vi "Constants.vi"() -> ()   [LabVIEW 2019, in "Reset Hardware Shared.lvlib"]
doc: "Use this Global VI to access the GUIDs assigned to the page resources of the Custom Device."
uses:
  Reset Hardware Shared.lvlib
panel:
  in  "Tab Control":enum32{"GUIDs", "Constants", "Properties"}(tab)
  in  "Reset Hardware":string="5e0dd9d5-b0d1-4b33-abc2-5f3c1ff7365d"
  in  "Reset XNET":string
  in  "Reset DAQmx AO":string
  in  "Compiled.Settings":string="Compiled.Settings"
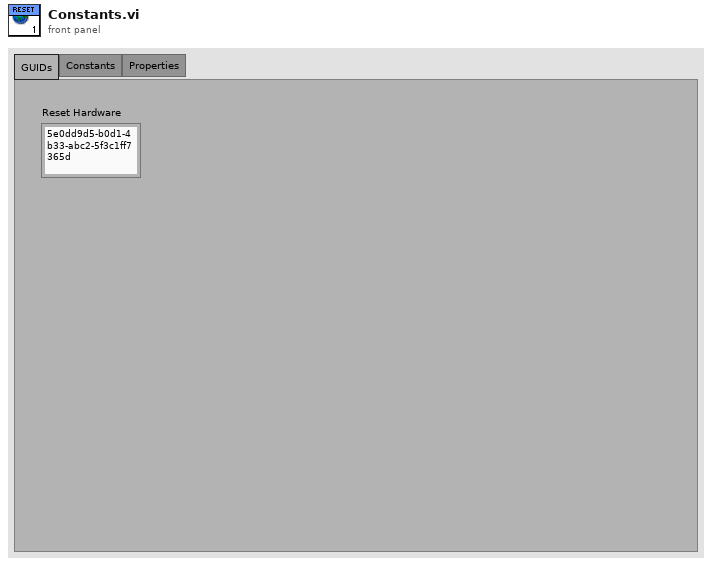
[diagram p1: front panel]
diagram:
